vi "Construct URI.vi"(6 "Arguments":cluster{"key":string, "value":string}[](array[cluster]), 8 "path":string, 9 "port":string, 10 "address":string, 11 "protocol":string) -> (3 "URI":string="opc.tcp://localhost:49580")   [LabVIEW 2013, in "URI.lvlib"]
uses:
  URI.lvlib
  <vilib>/regexp/Match Regular Expression.xnode
  <vilib>/wsapi/NI_WebServices.lvlib
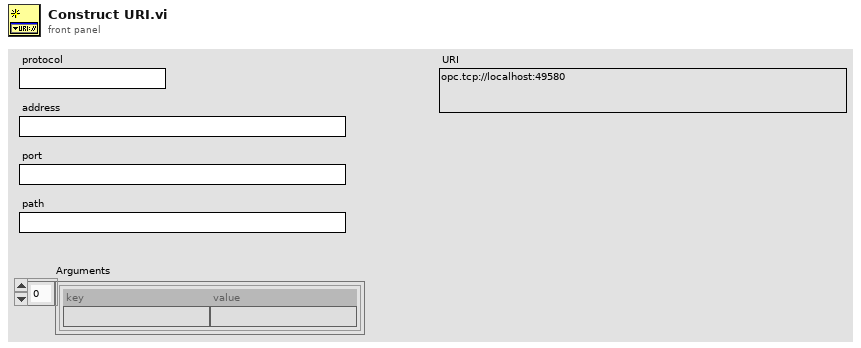
[diagram p1: front panel]
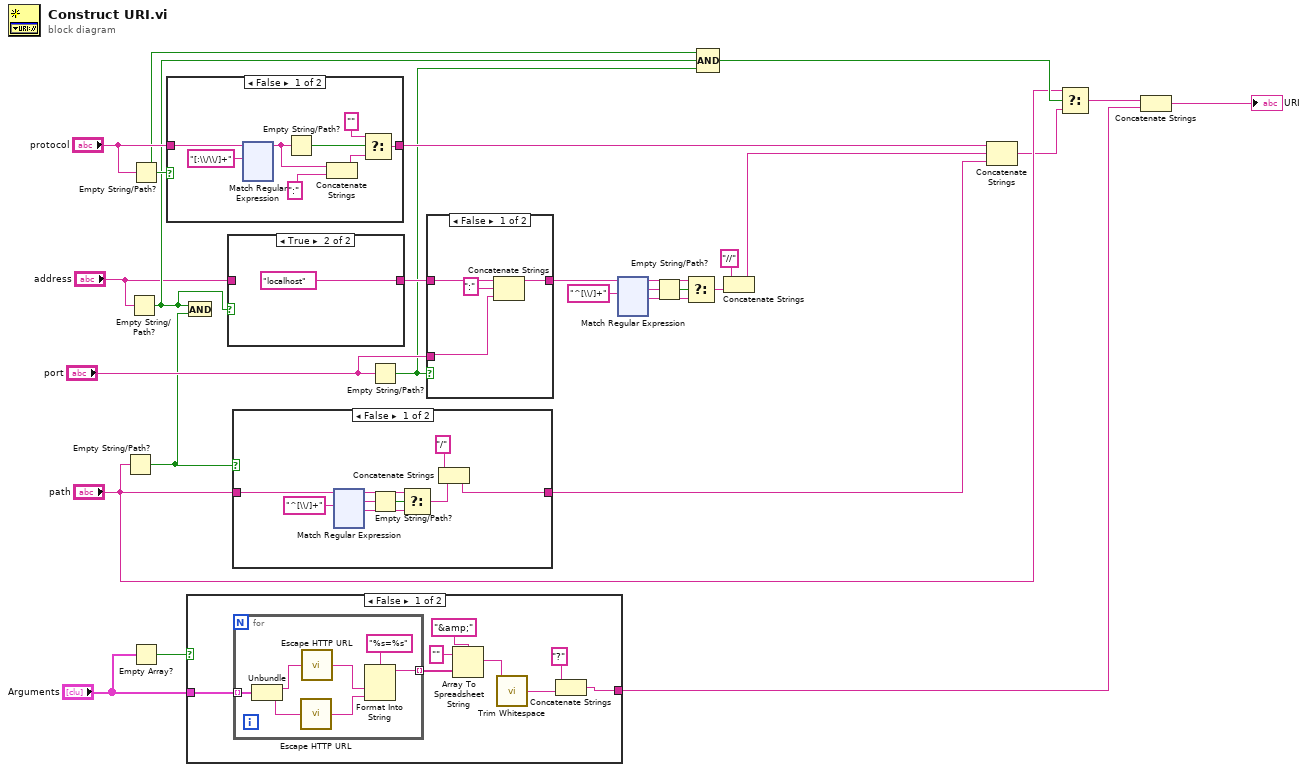
[diagram p0: block diagram]
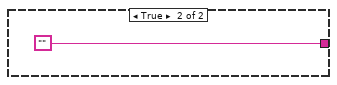
[diagram p2: hidden frame]
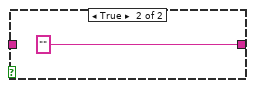
[diagram p6: hidden frame]
diagram:
  n1 = Empty String/Path?(string/path="path") -> (empty?=w22:bool)
  n2 = Empty String/Path?(string/path="address") -> (empty?=w16:bool)
  n3 = Empty String/Path?(string/path="protocol") -> (empty?=w21:bool)
  n4 = Empty Array?(array="Arguments") -> (empty?=w4:bool)
  n5 = case shown="False" w21 {
    tunnel: "protocol" -> [w34 _]
    tunnel: [w31 "" ("t")] -> w26
    frame False {
      n6 = xnode "Match Regular Expression"("input string"=w34, "regular expression"="[:\\/\\/]+") -> ("before match"=w29:string)  [unwired: 4 in, 4 out]
      n7 = Empty String/Path?(string/path=w29) -> (empty?=w33:bool)
      n8 = Concatenate Strings(w29, ":" ("t")) -> (w30:string)
      n9 = Select(t="", s=w33, f=w30) -> (s? t:f=w31:string)
    }
    frame True {
    }
  }
  n10 = And(x=w16, y=w22) -> ()  [unwired: 1 out]
  n11 = case shown="False" w4 {
    tunnel: "Arguments" -> [w158 _]
    tunnel: [w151 ""] -> w3
    frame False {
      n12 = for {
        tunnel: w158 -> [w165] mode=indexing
        tunnel: [w163] -> w157 mode=indexing
        n13 = Unbundle(w165) -> ("key"=w162:string, "value"=w160:string)
        n14 = call <vilib>:"Escape HTTP URL.vi"("unescaped string in"=w160) -> ("escaped string out"=w159:string)
        n15 = call <vilib>:"Escape HTTP URL.vi"("unescaped string in"=w162) -> ("escaped string out"=w161:string)
        n16 = Format Into String(format string="%s=%s", w161, w159) -> (resulting string=w163:string)  [unwired: 2 in, 1 out]
      }
      n17 = Array To Spreadsheet String(delimiter (Tab)="&amp;", array=w157, 3:"" ("format string")) -> (spreadsheet string=w154:string)
      n18 = call <vilib>:"Trim Whitespace.vi"("string"=w154) -> ("trimmed string"=w152:string)  [unwired: 1 in]
      n19 = Concatenate Strings("?" ("t"), w152) -> (w151:string)
    }
    frame True {
    }
  }
  n20 = case shown="True" w16 {
    tunnel: [w167 "localhost" ("t")] -> w24
    tunnel: "address" -> [w167 _]
    frame False {
    }
    frame True {
    }
  }
  n21 = case shown="False" w22 {
    tunnel: "path" -> [w170 w292]
    tunnel: [w176 w292] -> w23
    frame False {
      n22 = xnode "Match Regular Expression"("input string"=w170, "regular expression"="^[\\/]+") -> ("before match"=w173:string, "whole match"=w172:string, "after match"=w175:string)  [unwired: 4 in, 2 out]
      n23 = Empty String/Path?(string/path=w172) -> (empty?=w174:bool)
      n24 = Select(t=w173, s=w174, f=w175) -> (s? t:f=w169:string)
      n25 = Concatenate Strings("/" ("t"), w169) -> (w176:string)
    }
    frame True {
    }
  }
  n26 = Empty String/Path?(string/path="port") -> (empty?=w20:bool)
  n27 = case shown="False" w20 {
    tunnel: "port" -> [w293 _]
    tunnel: w24 -> [w296 w297]
    tunnel: [w295 w297] -> w8
    frame False {
      n28 = Concatenate Strings(w296, ":" ("t"), w293) -> (w295:string)
    }
    frame True {
    }
  }
  n29 = xnode "Match Regular Expression"("input string"=w8, "regular expression"="^[\\/]+") -> ("before match"=w11:string, "whole match"=w12:string, "after match"=w7:string)  [unwired: 4 in, 2 out]
  n30 = Empty String/Path?(string/path=w12) -> (empty?=w10:bool)
  n31 = Select(t=w11, s=w10, f=w7) -> (s? t:f=w9:string)
  n32 = Compound Arithmetic op=AND(w21, w16, w20) -> (w19:bool)
  n33 = Concatenate Strings("//" ("t"), w9) -> (w14:string)
  n34 = Concatenate Strings(w26, w14, w23) -> (w17:string)
  n35 = Select(t="path", s=w19, f=w17) -> (s? t:f=w2:string)
  n36 = Concatenate Strings(w2, w3) -> (→"URI":string)
